vi "h.SENSORS.AddSensor.vi"(4 "Sensor Calibration Factor":dbl=60.0, 5 "Instrument Channel":u32=1 min=1 max=16, 6 "Sensor Wavelength Band":T1=1550.0 items=["1470"=1470.0, "1490"=1490.0, "1510"=1510.0, "1530"=1530.0, "1550"=1550.0, "1570"=1570.0, "1590"=1590.0, "1610"=1610.0], 7 "error in":errorcluster, 8 "Sensor Model":string="os7510", 9 "Sensor Name":string="accel_1", 10 "Connection ID":refnum<k5>) -> (0 "error out":errorcluster, 3 "Connection ID Out":refnum<k5>)   [LabVIEW 2016, in "h.Library.lvlib"]
uses:
  h.Library.lvlib
  h.SENSORS.FPFilterBands.ctl
panel:
  in  "Distance":i32=1
  out "Message":string
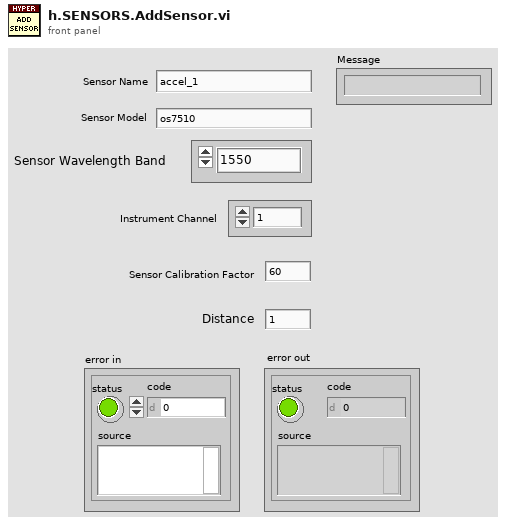
[diagram p1: front panel]
types:
  T1 = typedef "h.Library.lvlib/h.SENSORS.FPFilterBands.ctl" = dbl
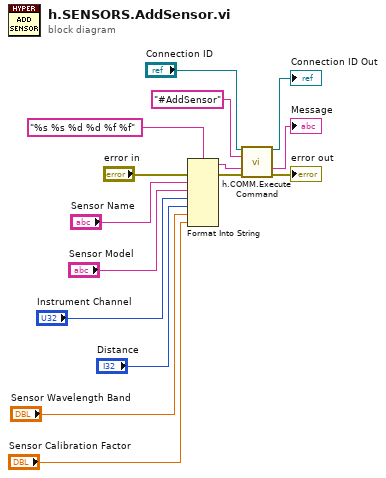
[diagram p0: block diagram]
diagram:
  n1 = Format Into String(format string="%s %s %d %d %f %f", error in="error in", "Sensor Name", "Sensor Model", "Instrument Channel", "Distance", "Sensor Wavelength Band", "Sensor Calibration Factor") -> (resulting string=w1:string, error out=w9:errorcluster)  [unwired: 1 in]
  n2 = call "h.COMM.Execute Command.vi"("Connection ID"="Connection ID", "Command"="#AddSensor", "Argument"=w1, "error in"=w9) -> ("Connection ID out"=→"Connection ID Out":refnum<k5>, "Message"=→"Message":string, "error out"=→"error out":errorcluster)  [unwired: 4 in, 5 out]
